vi "Eat.vi"(8 "error in (no error)":errorcluster, 10 "String":string, 11 "Cow in":refnum<class "Cow.lvclass">) -> (0 "error out":errorcluster, 2 "String 2":string, 3 "Cow out":refnum<class "Cow.lvclass">)   [LabVIEW 2018, in "Cow.lvclass"]
uses:
  Cow.lvclass
  animal/Animal.lvclass
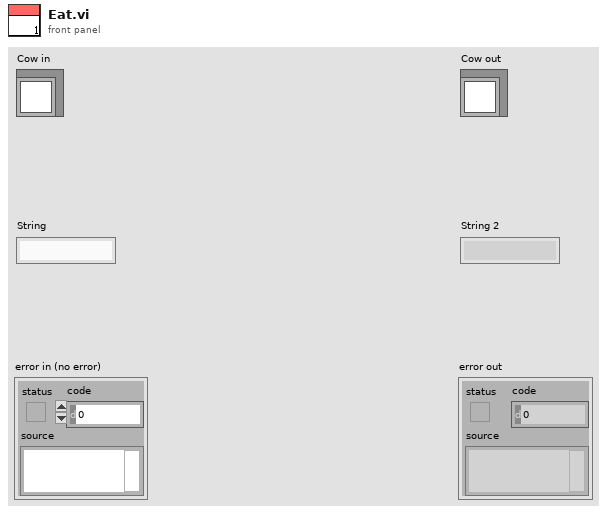
[diagram p1: front panel]
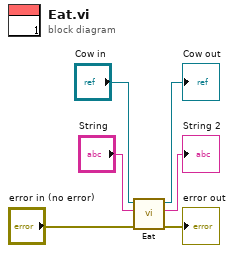
[diagram p0: block diagram]
diagram:
  n1 = call-parent "Eat.vi"("error in (no error)"="error in (no error)", "String"="String", "Animal in"="Cow in") -> ("error out"=→"error out":errorcluster, "String 2"=→"String 2":string, "Animal out"=→"Cow out":refnum<class "Cow.lvclass">)  [unwired: 6 in]
